vi "@create.vi"(6 "autorun? (false)":bool, 7 "dotnet_system_exec in":refnum<class "dotnet_system_exec.lvclass">, 8 "error in (no error)":errorcluster, 9 "working directory (c:\\)":path=path "c:/", 10 "arguments (\"\")":string, 11 "command line (cmd.exe)":string="cmd.exe") -> (0 "error out":errorcluster, 2 "public events":T1, 3 "dotnet_system_exec out":refnum<class "dotnet_system_exec.lvclass">)   [LabVIEW 2015, in "dotnet_system_exec.lvclass"]
doc: "Creates an instance of the .NET System Process. It configures the instance not to show a window but to redirect the stdout, stderr, and stdin so that LabVIEW can interface with them. Use the public events to register for the stdout and stderr events."
uses:
  dotnet_system_exec.lvclass
  dotnet_system_exec.lvclass/dotnet_system_exec.ctl
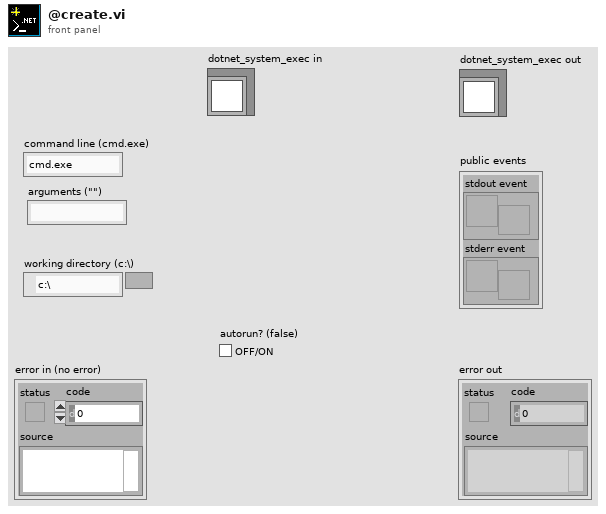
[diagram p1: front panel]
types:
  T1 = cluster{"stdout event":refnum<user-event>, "stderr event":refnum<user-event>}
  T2 = cluster{"StdOut Event":refnum<user-event>, "StdErr Event":refnum<user-event>}
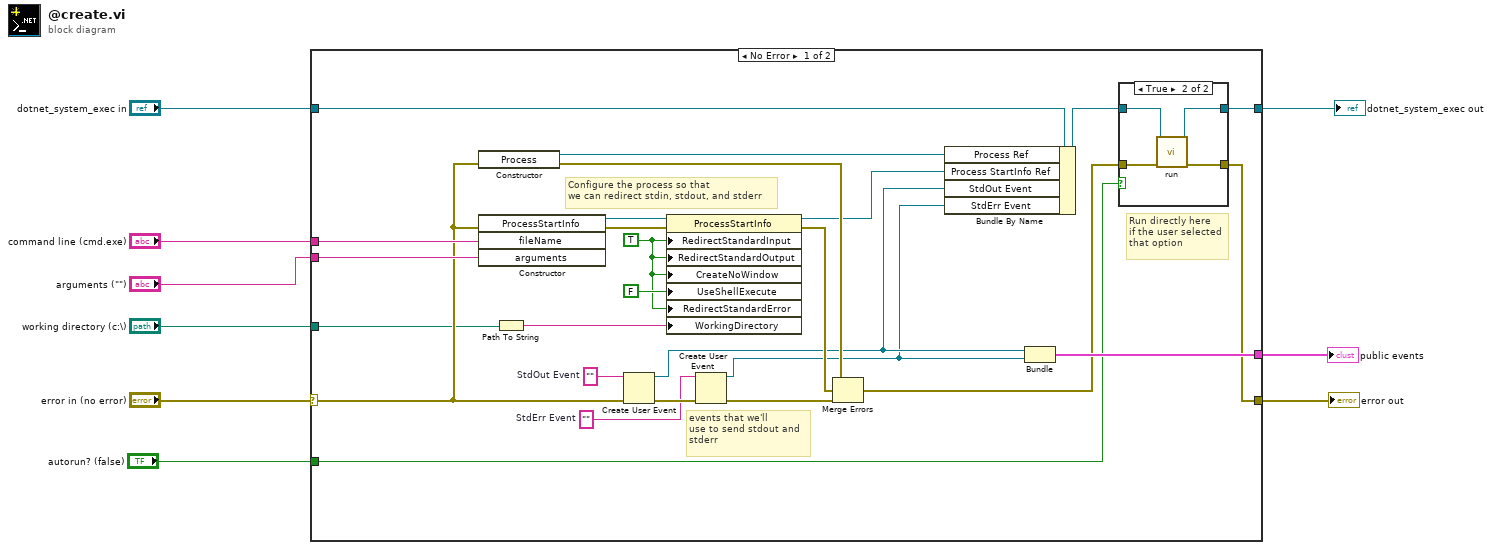
[diagram p0: block diagram]
diagram:
  n1 = case shown="No Error" "error in (no error)" {
    selector: "error in (no error)" -> [w19 w43]
    tunnel: [w11 w43] -> w8
    tunnel: [w13 w42] -> w6
    tunnel: "dotnet_system_exec in" -> [w26 w42]
    tunnel: "command line (cmd.exe)" -> [w29 _]
    tunnel: "arguments (\"\")" -> [w28 _]
    tunnel: "working directory (c:\\)" -> [w15 _]
    tunnel: [w18 _] -> w2
    tunnel: "autorun? (false)" -> [w10 _]
    frame No Error {
      w21 = ""  # StdErr Event
      w23 = ""  # StdOut Event
      w32 = TRUE ("RedirectStandardInput")
      # "Configure the process so that\nwe can redirect stdin, stdout, and stderr"
      # "events that we'll\nuse to send stdout and\nstderr"
      # "Run directly here\nif the user selected\nthat option"
      n2 = constructor class="Process"(error in=w19) -> (reference out=w25:refnum<k24>, error out=w31:errorcluster)  [unwired: 2 in, 1 out]
      n3 = constructor class="ProcessStartInfo"(error in=w19, "fileName"=w29, "arguments"=w28) -> (reference out=w34:refnum<k24>, error out=w35:errorcluster)  [unwired: 2 in, 3 out]
      n4 = Path To String(path=w15) -> (string=w27:string)
      n5 = Create User Event(user event datatype=w23, error in=w19) -> (user event=w17:refnum<user-event>, error out=w22:errorcluster)
      n6 = property class="ProcessStartInfo"(reference=w34, error in=w35, "RedirectStandardInput"=w32, "RedirectStandardOutput"=w32, "CreateNoWindow"=w32, "UseShellExecute"=FALSE, "RedirectStandardError"=w32, "WorkingDirectory"=w27) -> (reference out=w24:refnum<k24>, error out=w30:errorcluster)
      n7 = Create User Event(user event datatype=w21, error in=w22) -> (user event=w16:refnum<user-event>, error out=w20:errorcluster)
      n8 = Merge Errors(w31, w30, w20) -> (w12:errorcluster)
      n9 = Bundle By Name(cluster=w26, "Process Ref"=w25, "Process StartInfo Ref"=w24, "StdOut Event"=w17, "StdErr Event"=w16) -> (w14:refnum<class "dotnet_system_exec.lvclass">)
      n10 = Bundle("StdOut Event"=w17, "StdErr Event"=w16) -> (w18:T2)  [unwired: 1 in]
      n11 = case shown="True" w10 {
        tunnel: w14 -> [w37 w41]
        tunnel: [w37 w40] -> w13
        tunnel: w12 -> [w36 w39]
        tunnel: [w36 w38] -> w11
        frame False {
        }
        frame True {
          n12 = call "run.vi"("error in (no error)"=w39, "dotnet_system_exec in"=w41) -> ("error out"=w38:errorcluster, "dotnet_system_exec out"=w40:refnum<class "dotnet_system_exec.lvclass">)  [unwired: 8 in]
        }
      }
    }
    frame Error {
    }
  }
  "error out" <- w8
  "dotnet_system_exec out" <- w6
  "public events" <- w2
